vi "Arttu_v09_1.vi"() -> ()   [LabVIEW 2015]
panel:
  out "element":bool
  out "Started:":string
  in  "SHUTDOWN":bool
  in  "MASTER CONTROL":bool
  in  "Tab Control":T1(tab)
  in  "Read Seq":bool
  in  "Save Seq":bool
  in  "Configuration file":path=path "C:/Users/shresplab/Desktop/BerttaConfiguration.lvm" caption="Filename"
  in  "OK Button 2":bool
  out "Boolean":bool
  in  "User (initials)":string
  in  "Project name":string
  in  "Description":string
  out "Output file":string
  out "PUMP 3":bool
  out "Target amount":dbl
  out "Scale weight":dbl
  out "Amount now":dbl
  out "Flow rate":dbl
  out "Time to target":dbl format="%<%H:%M:%S>t"
  out "Current step":dbl
  out "Target amount":dbl
  out "Amount now":dbl
  out "Amount now":dbl
  out "Target amount":dbl
  out "Current step":dbl
  out "Time to target":dbl format="%<%H:%M:%S>t"
  out "Flow rate":dbl
  out "Amount now":dbl
  out "Scale weight":dbl
  out "Target amount":dbl
  out "PUMP 2":bool
  out "Sensor OK 6":bool
  out "Sensor OK 5":bool
  out "Sensor OK 4":bool
  out "Sensor OK 3":bool
  in  "OK Button":bool
  in  "Add comment":string
  out "PUMP 1":bool
  out "Target amount":dbl
  out "Scale weight":dbl
  out "Amount now":dbl
  out "Flow rate":dbl
  out "Time to target":dbl format="%<%H:%M:%S>t"
  out "Current step":dbl
  out "Target amount":dbl
  out "Amount now":dbl
  out "Tr":dbl
  out "Tj in":dbl
  out "Tj out":dbl
  out "T set":dbl
  out "Current step":i32
  out "RPM":dbl
  out "Torque 2":dbl
  out "Waveform Chart 5":dynamicdata(graph)
  out "Waveform Chart 6":dynamicdata(graph)
  out "Waveform Chart 7":dynamicdata(graph)
  in  "Tab Control 2":T2(tab)
  out "Waveform Chart 3":dynamicdata(graph)
  out "Waveform Chart 8":dynamicdata(graph)
  out "Waveform Chart 11":dynamicdata(graph)
  out "Waveform Chart 13":dynamicdata(graph)
  out "Waveform Chart 9":dynamicdata(graph)
  out "Table":string[][](table)=[["14.8.2017 18.06.59", "0,000000", "417,670000", "-0,150000", "1,000000", "22,220000", "23,366837", "23,574959", "23,985852", "23,690000", "240,000000", "4,000000", "0,000000", "397,000000", "-397,000000", "1,000000"], ["14.8.2017 18.07.06", "0,000000", "417,640000", "-0,120000", "1,000000", "22,220000", "23,763115", "23,906257", "23,985694", "23,680000", "240,000000", "4,000000", "0,000000", "397,000000", "-397,000000", "1,000000"], ["14.8.2017 18.07.13", "0,000000", "417,640000", "-0,120000", "1,000000", "22,220000", "23,965922", "24,013440", "23,984906", "23,670000", "240,000000", "4,100000", "3,000000", "397,000000", "-397,000000", "1,000000"], ["14.8.2017 18.07.21", "0,000000", "417,640000", "-0,120000", "1,000000", "22,220000", "23,943860", "23,900110", "23,987113", "23,670000", "240,000000", "4,000000", "0,000000", "397,000000", "-397,000000", "1,000000"], ["14.8.2017 18.07.28", "0,000000", "417,640000", "-0,120000", "1,000000", "22,220000", "23,736328", "23,600018", "23,989004", "23,660000", "240,000000", "4,000000", "0,000000", "397,000000", "-397,000000", "1,000000"], ["14.8.2017 18.07.36", "0,000000", "417,640000", "-0,120000", "1,000000", "22,220000", "23,480910", "23,324538", "23,991053", "23,660000", "240,000000", "4,000000", "0,000000", "397,000000", "-397,000000", "1,000000"], ["14.8.2017 18.07.43", "0,000000", "417,640000", "-0,120000", "2,000000", "22,220000", "23,195579", "23,008270", "23,999093", "23,650000", "240,000000", "4,000000", "0,000000", "397,000000", "-397,000000", "1,000000"], ["14.8.2017 18.07.51", "0,000000", "417,650000", "-417,650000", "1,000000", "22,220000", "22,862541", "22,649021", "24,003979", "23,650000", "240,000000", "4,000000", "0,000000", "397,000000", "-397,000000", "2,000000"], ["14.8.2017 18.07.58", "0,000000", "417,640000", "0,010000", "1,000000", "22,220000", "22,541353", "22,354878", "24,005398", "23,650000", "240,000000", "4,000000", "0,000000", "397,000000", "-397,000000", "1,000000"], ["14.8.2017 18.08.06", "0,000000", "417,640000", "0,010000", "1,000000", "22,220000", "22,347931", "22,253738", "24,007605", "23,640000", "240,000000", "4,100000", "0,000000", "397,000000", "-397,000000", "1,000000"], ["14.8.2017 18.08.13", "0,000000", "417,640000", "0,010000", "1,000000", "22,220000", "22,329030", "22,302102", "24,006028", "23,640000", "240,000000", "4,000000", "0,000000", "395,820000", "-395,820000", "1,000000"], ["14.8.2017 18.08.20", "0,000000", "417,640000", "0,010000", "1,000000", "22,220000", "22,466849", "22,511320", "24,002403", "23,630000", "240,000000", "4,000000", "0,000000", "395,830000", "-0,010000", "1,000000"], ["14.8.2017 18.08.28", "0,000000", "417,640000", "0,010000", "1,000000", "22,220000", "22,707062", "22,835101", "24,000984", "23,620000", "240,000000", "4,000000", "0,000000", "395,830000", "-0,010000", "1,000000"], ["14.8.2017 18.08.35", "0,000000", "417,640000", "0,010000", "1,000000", "22,220000", "23,054104", "23,232979", "24,001299", "23,600000", "240,000000", "4,000000", "0,000000", "395,830000", "-0,010000", "1,000000"], ["14.8.2017 18.08.43", "0,000000", "417,640000", "0,010000", "1,000000", "22,220000", "23,412371", "23,522793", "24,002560", "23,590000", "240,000000", "4,000000", "0,000000", "395,820000", "0,000000", "1,000000"], ["14.8.2017 18.08.51", "0,000000", "417,640000", "0,010000", "1,000000", "22,220000", "23,596247", "23,656125", "24,003821", "23,580000", "240,000000", "4,000000", "0,000000", "395,820000", "0,000000", "1,000000"]]
  in  "T ext / T ext 2":enum32{"External 1", "External 2"}(radio)
  out "Sensor OK":bool
  in  "T fail":dbl=20.0
  out "Boolean 12":bool
  out "Boolean 7":bool
  out "Boolean 6":bool
  out "Boolean 5":bool
  out "Boolean 4":bool
  in  "?":bool
  in  "T manual setpoint":dbl=20.0
  in  "Lauda port":dbl=9.0
  in  "Manual select":enum32{"Tr", "Tj"}(radio)
  in  "TempSeq":dbl[][](array[numeric])=[[20.0, 20.0, 0.0, 20.0], [20.0, 20.0, 0.0, 20.0], [50.0, 20.0, 0.0, 20.0], [20.0, 20.0, 0.0, 20.0], [20.0, 20.0, 0.0, 20.0], [20.0, 20.0, 1000.0, 20.0]]
  out "T control":dbl
  out "Tr":dbl
  out "Tj in":dbl
  out "Tj out":dbl
  out "DT":dbl
  out "Elapsed":i32 format="%<%H:%M:%S>T"
  in  "PAUSE":bool
  out "Boolean 19":bool
  in  "Reset":bool
  in  "Treshold (Tset)":dbl=1.0
  in  "Tmax":dbl=199.0
  in  "Tmin":dbl=20.0
  out "Waveform Chart":dynamicdata(graph)
  out "T external 2":dbl
  in  "Xe":dbl=1.0
  in  "Port":i32=10
  in  "Radio Buttons 3":enum32{"Reglo Digital", "Reglo Analog", "PAM"}(radio)=enum."Reglo Analog"
  out "Speed":dbl
  out "mA":dbl format="%#_2g"
  in  "Port":i32=15
  out "RPM":dbl format="%#_2g"
  out "Led10 3":bool
  out "Led9 3":bool
  out "Led8 3":bool
  out "Led7 3":bool
  out "Led6 3":bool
  out "Led5 3":bool
  out "Led4 3":bool
  out "Led3 3":bool
  out "Led2 3":bool
  out "Led1 3":bool
  in  "PumpSeq 3":dbl[][](array[numeric])=[[0.0, 0.0, 7.0], [0.0, 0.0, 2.0], [0.0, 0.0, 100.0], [0.0, 0.0, 0.0], [0.0, 0.0, 0.0], [0.0, 0.0, 0.0], [0.0, 0.0, 0.0], [0.0, 0.0, 0.0], [0.0, 0.0, 0.0], [0.0, 0.0, 0.0], [0.0, 1.0, 0.0]]
  in  "?":bool
  out "Flow rate (g/min)":dbl
  out "Scale reading":dbl
  out "Step amount now":dbl
  out "Time to target":dbl format="%<%H:%M:%S>t"
  in  "Grams / min":dbl
  out "Waveform Chart 12":dynamicdata(graph)
  in  "?":bool
  out "Total amount now":dbl
  out "Total time 3":dbl
  out "Total amount target 3":dbl
  out "Led11 3":bool
  in  "Reset 4":bool
  in  "Port":i32=11
  in  "Radio Buttons 2":enum32{"Reglo Digital", "Reglo Analog", "PAM"}(radio)
  out "Speed":dbl
  out "mA":dbl format="%#_2g"
  in  "Port":i32=15
  out "RPM":dbl format="%#_2g"
  out "Led10 2":bool
  out "Led9 2":bool
  out "Led8 2":bool
  out "Led7 2":bool
  out "Led6 2":bool
  out "Led5 2":bool
  out "Led4 2":bool
  out "Led3 2":bool
  out "Led2 2":bool
  out "Led1 2":bool
  in  "PumpSeq 2":dbl[][](array[numeric])=[[0.0, 0.0, 7.0], [0.0, 0.0, 2.0], [0.0, 0.0, 100.0], [0.0, 0.0, 0.0], [0.0, 0.0, 0.0], [0.0, 0.0, 0.0], [0.0, 0.0, 0.0], [0.0, 0.0, 0.0], [0.0, 0.0, 0.0], [0.0, 0.0, 0.0], [0.0, 1.0, 0.0]]
  in  "?":bool
  out "Flow rate (g/min)":dbl
  out "Scale reading":dbl
  out "Step amount now":dbl
  out "Time to target":dbl format="%<%H:%M:%S>t"
  in  "Grams / min":dbl
  out "Waveform Chart 10":dynamicdata(graph)
  in  "?":bool
  out "Total amount now":dbl
  out "Total time 2":dbl
  out "Total amount target 2":dbl
  out "Led11 2":bool
  in  "Reset 3":bool
  in  "Port":i32=12
  in  "Radio Buttons":enum32{"Reglo Digital", "Reglo Analog", "PAM"}(radio)
  out "Speed":dbl
  out "mA":dbl format="%#_2g"
  in  "Port":i32=14
  out "RPM":dbl format="%#_2g"
  out "Led10":bool
  out "Led9":bool
  out "Led8":bool
  out "Led7":bool
  out "Led6":bool
  out "Led5":bool
  out "Led4":bool
  out "Led3":bool
  out "Led2":bool
  out "Led1":bool
  in  "PumpSeq":dbl[][](array[numeric])=[[0.0, 0.0, 7.0], [0.0, 0.0, 2.0], [0.0, 0.0, 100.0], [0.0, 0.0, 0.0], [0.0, 0.0, 0.0], [0.0, 0.0, 0.0], [0.0, 0.0, 0.0], [0.0, 0.0, 0.0], [0.0, 0.0, 0.0], [0.0, 0.0, 0.0], [0.0, 1.0, 0.0]]
  in  "?":bool
  out "Flow rate (g/min)":dbl
  out "Scale reading":dbl
  out "Step amount now":dbl
  out "Time to target":dbl format="%<%H:%M:%S>t"
  in  "Grams / min":dbl
  out "Waveform Chart 2":dynamicdata(graph)
  in  "?":bool
  out "Total amount now":dbl
  out "Total time":dbl
  out "Total amount target":dbl
  out "Led11":bool
  in  "Reset 2":bool
  in  "Bypass select 2":enum32{"Remote", "Manual"}(radio)
  in  "Port":dbl=13.0
  out "RPM":dbl
  out "Torque":dbl
  in  "Set RPM":dbl(slide) scale=0.0..500.0
  out "Waveform Chart 4":dynamicdata(graph)
  in  "Adjust T":dbl
  in  "Cal pump 3":dbl=1.11
  in  "Cal pump 2":dbl=1.218 format="%#_13g"
  in  "Cal pump 1":dbl=1.0 format="%#_13g"
  out "DAQ 9217 (PT100)":errorcluster
  # "Temperature sensor:"
  # "Manual control:"
  # "PUMP & SCALE 1"
  # "STEP"
  # "TOTAL"
  # "PUMP & SCALE 2"
  # "STEP"
  # "TOTAL"
  # "PUMP & SCALE 3"
  # "STEP"
  # "TOTAL"
  # "Tinit     >    Tset          Wait            Tfail"
  # "Manual control / end of sequence"
  # "Manual control"
  # "Secondary temperature sensor"
  # "Device communication"
  # "Grams    /   min"
  # "End of sequence"
  # "Manual control"
  # "Device communication"
  # "Pump configuration"
  # "Scale configuration"
  # "SCALE 1"
  # "Grams    /   min"
  # "End of sequence"
  # "Manual control"
  # "Device communication"
  # "Pump configuration"
  # "Scale configuration"
  # "SCALE 2"
  # "Grams    /   min"
  # "End of sequence"
  # "Manual control"
  # "Device communication"
  # "Pump configuration"
  # "Scale configuration"
  # "SCALE 3"
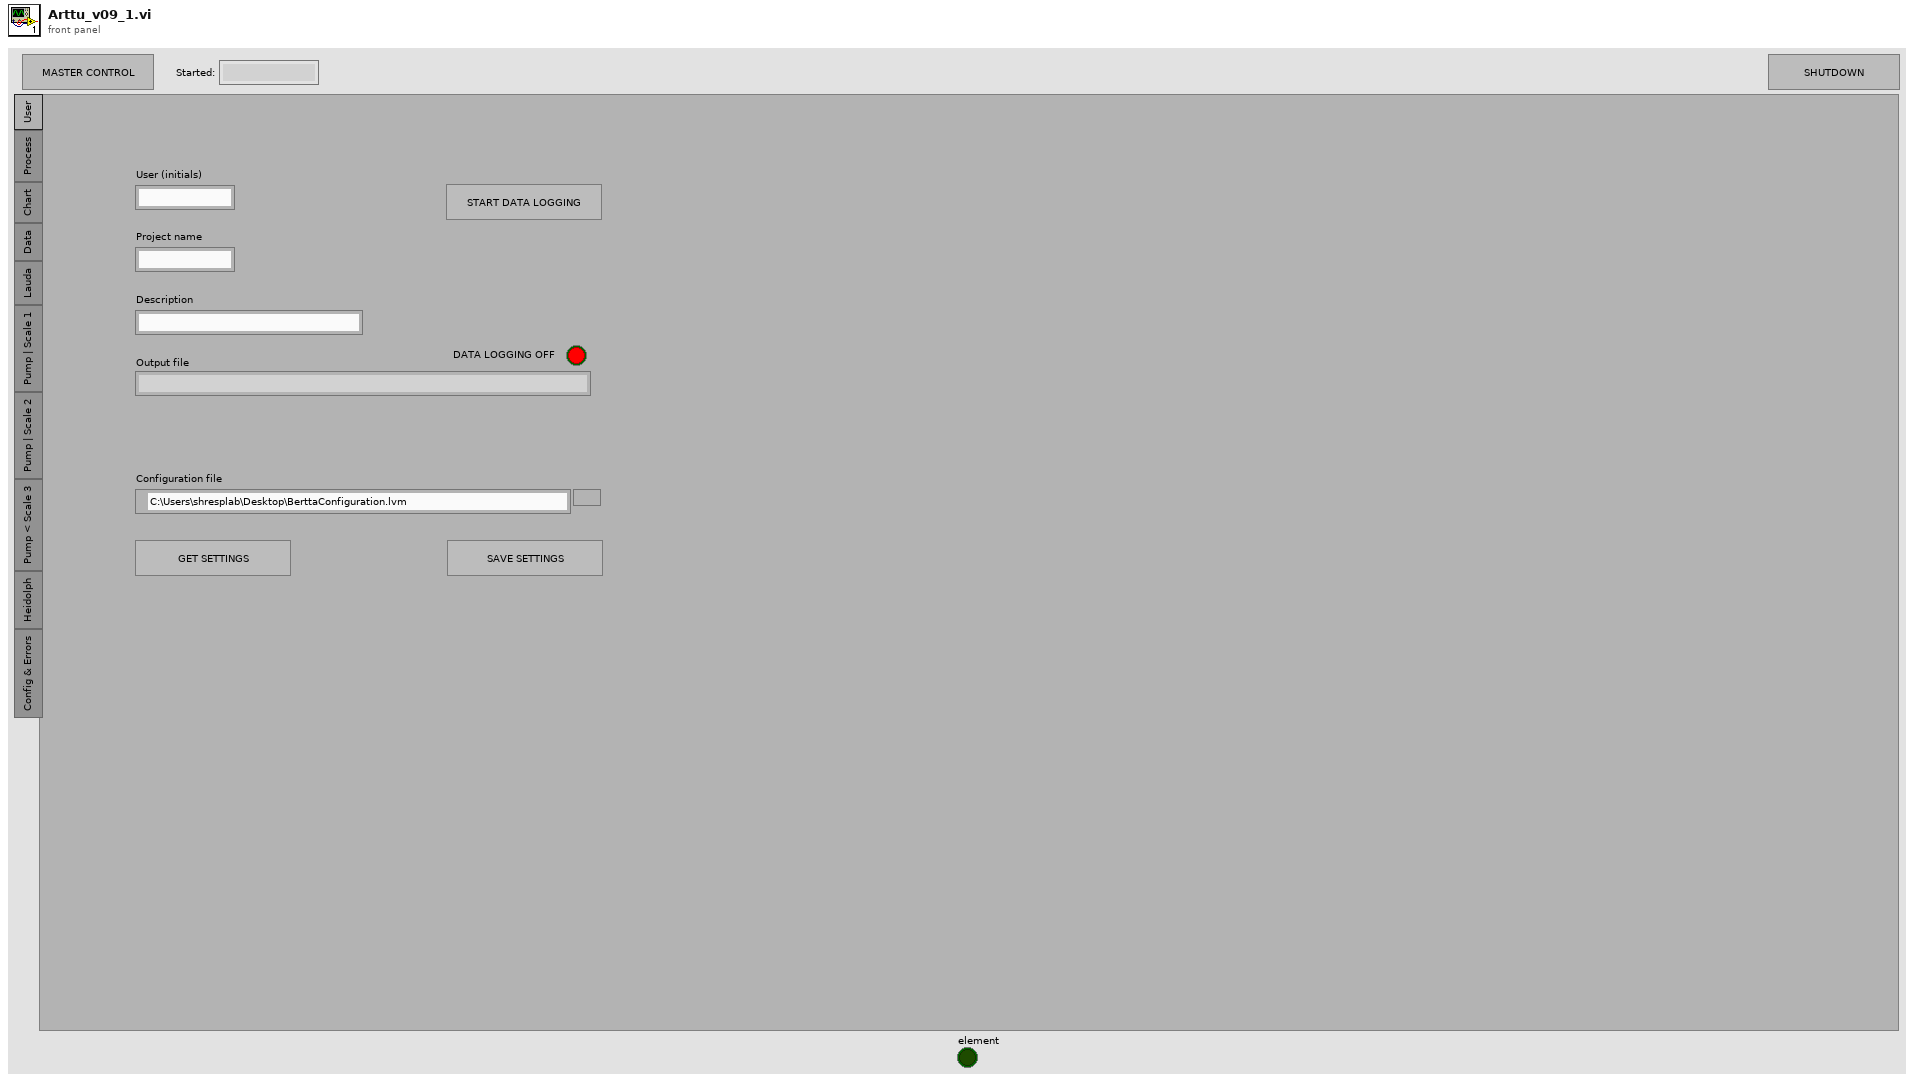
[diagram p1: front panel]
types:
  T1 = enum32{"User", "Process", "Chart", "Data", "Lauda", "Pump | Scale 1", "Pump | Scale 2", "Pump < Scale 3", "Heidolph", "Config & Errors"}
  T2 = enum32{"Temperatures", "Scale / Pump 1", "Scale / Pump 2", "Scale / Pump 3", "RPM / torque"}
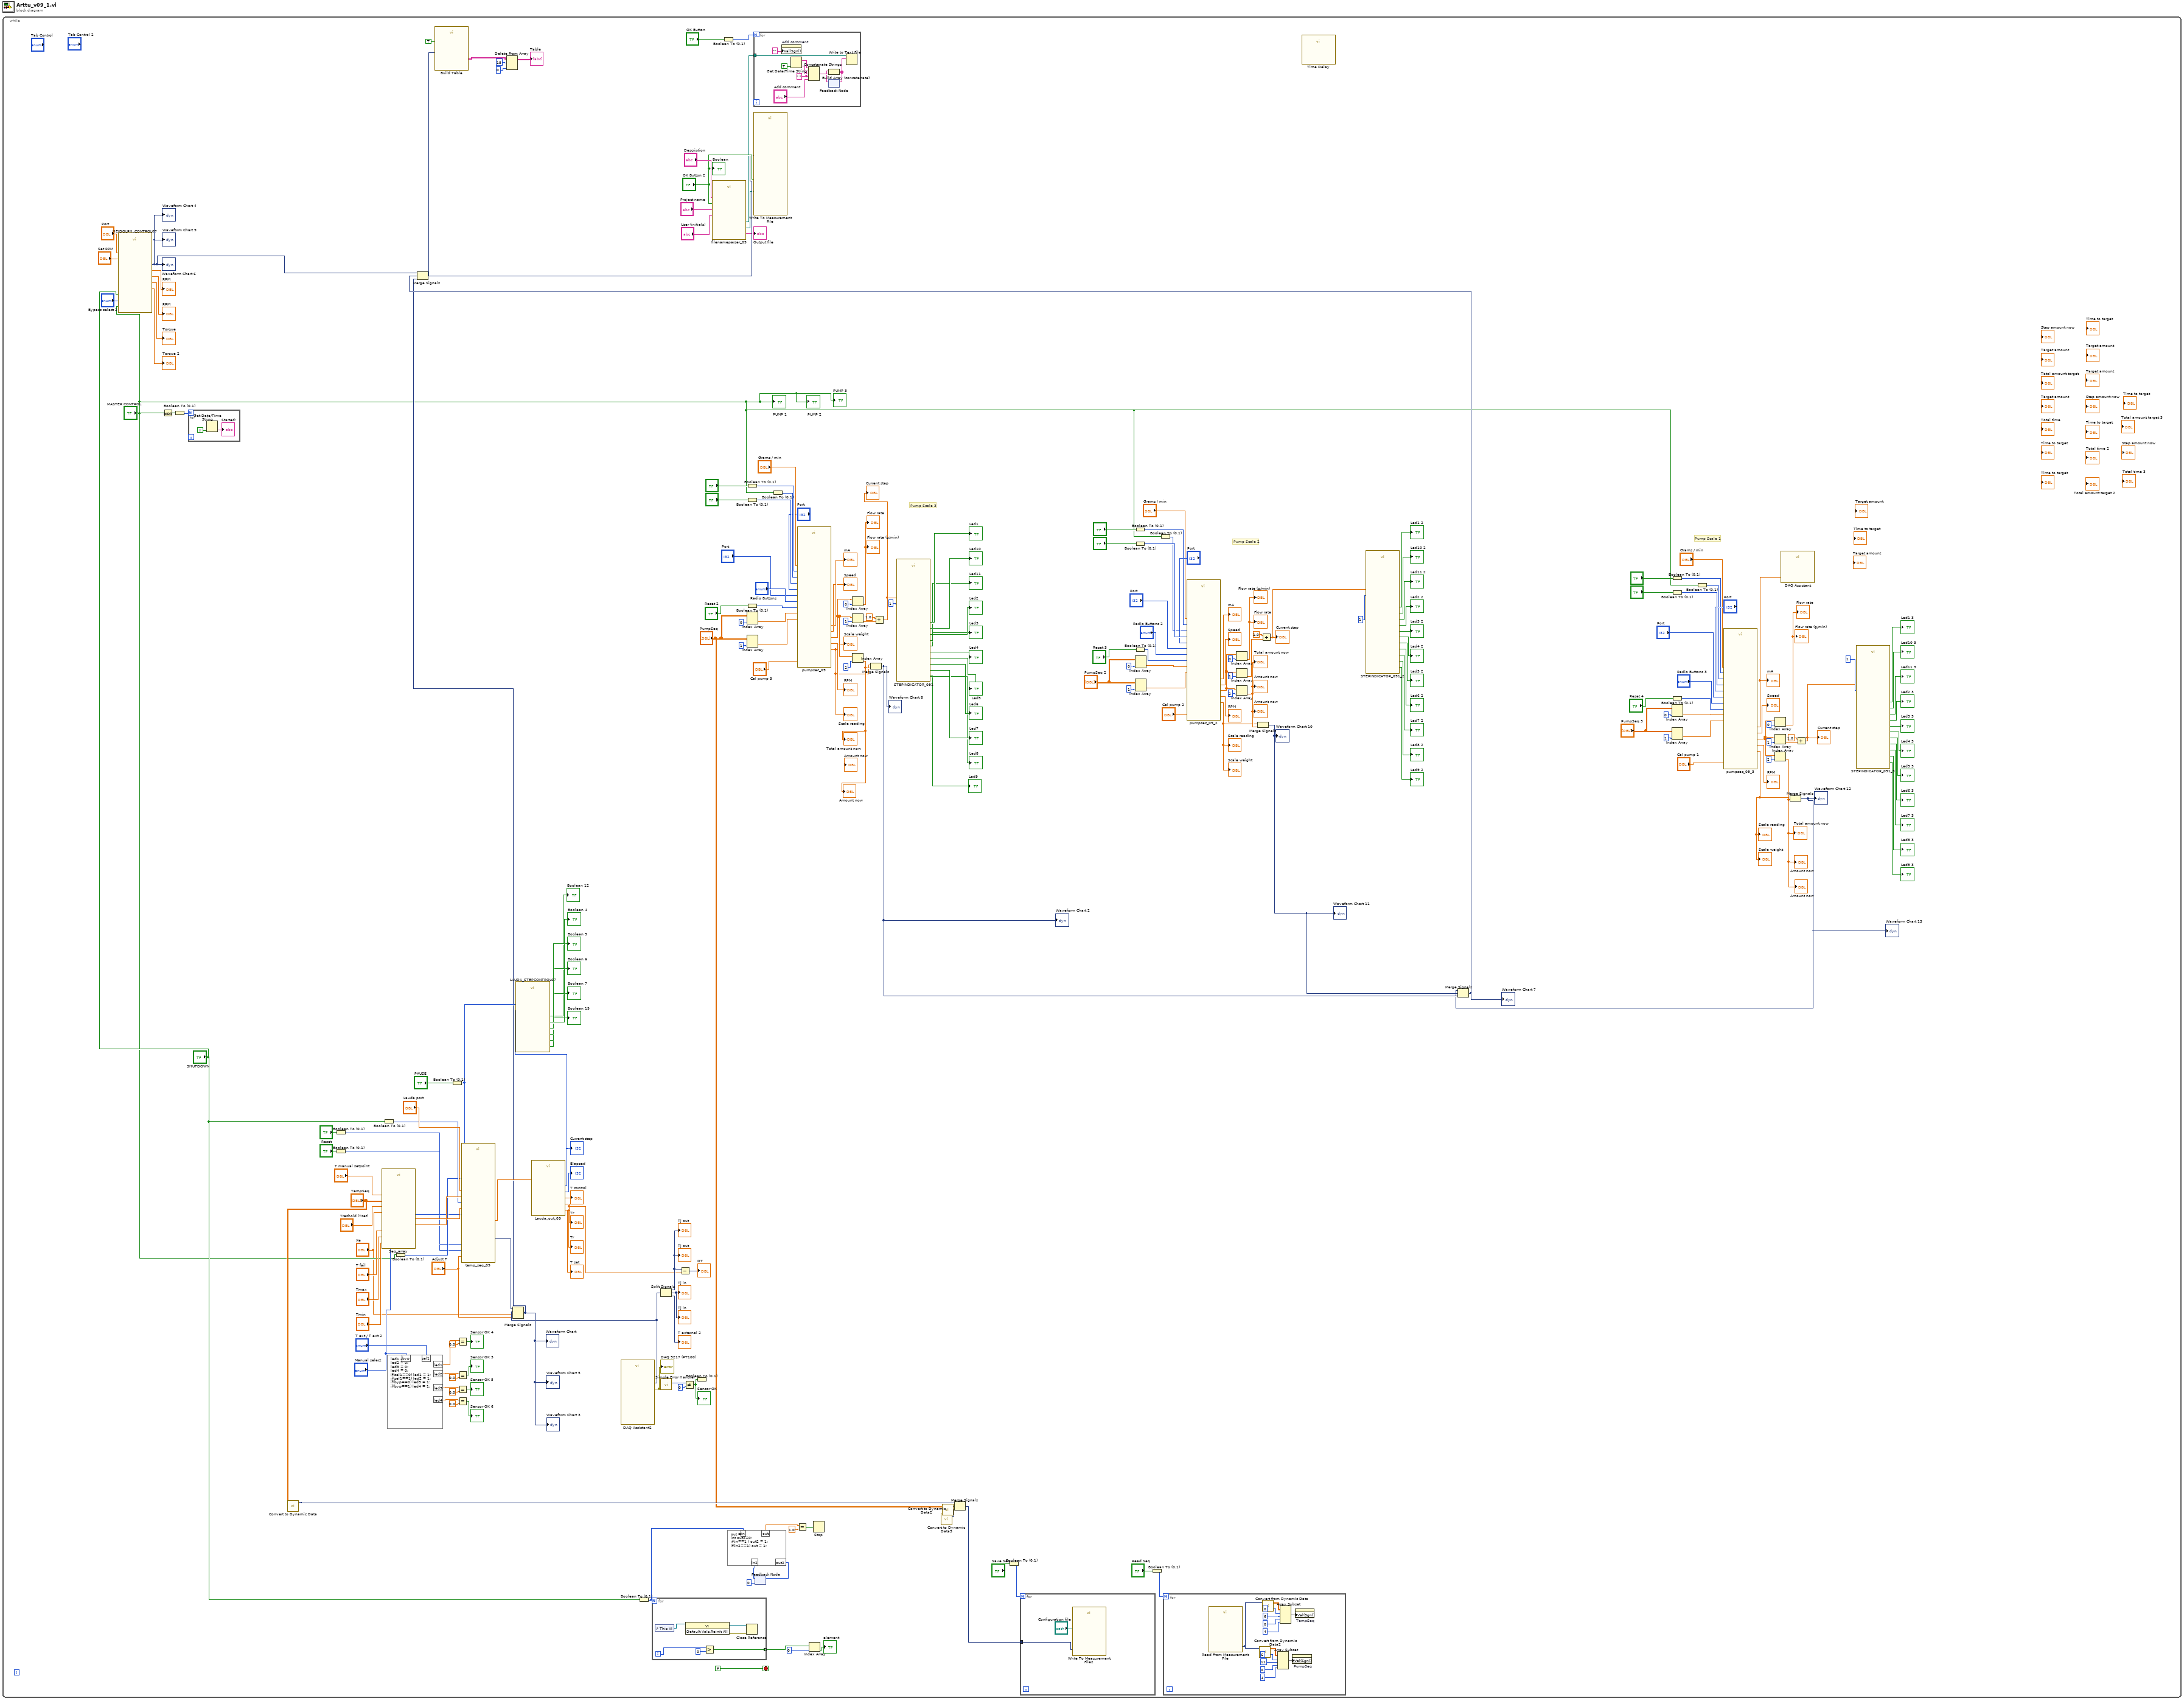
[diagram p0: block diagram]
diagram:
  n1 = while {
    stop <- FALSE stop-if-true
    # "Pump Scale 3"
    # "Pump Scale 2"
    # "Pump Scale 1"
    n2 = call "HEIDOLPH_CONTROL07.vi"("master"="MASTER CONTROL", "shutdown"="SHUTDOWN", "Bypass select"="Bypass select 2", "Set RPM"="Set RPM", "Device port"="Port") -> ("Dynamic Data"=w226:dynamicdata, "RPM"=→"RPM":dbl, "RPM 2"=→"RPM":dbl, "Torque"=→"Torque":dbl, "Torque 2"=→"Torque 2":dbl)  [unwired: 2 in]
    "Waveform Chart 4" <- w226
    "Waveform Chart 6" <- w226
    "Waveform Chart 9" <- w226
    n3 = Not(x="MASTER CONTROL") -> (.not. x?=w211:bool)
    n4 = Boolean To (0,1)(Boolean=w211) -> (0, 1=w212:i16)
    n5 = for {
      N: w212 -> [_]
      n6 = Get Date/Time String(want seconds? (F)=TRUE) -> (time string=→"Started:":string)  [unwired: 2 in, 1 out]
    }
    n7 = call "Convert to Dynamic Data"("2D Array"="TempSeq") -> ("Dynamic Data Type"=w208:dynamicdata)  [unwired: 3 in]
    n8 = Boolean To (0,1)(Boolean="Reset") -> (0, 1=w150:i16)
    n9 = Boolean To (0,1)(Boolean="?") -> (0, 1=w152:i16)
    n10 = call "Seq_array.vi"("Tfail_manual"="T fail", "TempSeq in"="TempSeq", "Tmin"="Tmin", "Tmax"="Tmax", "Treshold (Tset)"="Treshold (Tset)", "T manual setpoint"="T manual setpoint", "Xe"="Xe") -> ("TimeParams"=w164:dbl[], "TempParams"=w165:dbl[])  [unwired: 3 in]
    n11 = Boolean To (0,1)(Boolean="SHUTDOWN") -> (0, 1=w160:i16)
    n12 = formula code="led1 = 0;\nled2 = 0;\nled3 = 0;\nled4 = 0;\nif(sel1==0) led1 = 1;\nif(sel1==1) led2 = 1;\nif(byp==0) led3 = 1;\nif(byp==1) led4 = 1;"("sel1"="T ext / T ext 2", "byp"="Manual select") -> ("led1"=w179:dbl, "led2"=w177:dbl, "led3"=w172:dbl, "led4"=w171:dbl)
    n13 = Boolean To (0,1)(Boolean="MASTER CONTROL") -> (0, 1=w159:i16)
    n14 = Boolean To (0,1)(Boolean="PAUSE") -> (0, 1=w156:i16)
    n15 = Equal?(x=w179, y=0.0) -> (x = y?=→"Sensor OK 4":bool)
    n16 = Equal?(x=w177, y=0.0) -> (x = y?=→"Sensor OK 3":bool)
    n17 = Equal?(x=w172, y=0.0) -> (x = y?=→"Sensor OK 5":bool)
    n18 = Equal?(x=w171, y=0.0) -> (x = y?=→"Sensor OK 6":bool)
    n19 = call "temp_seq_09.vi"("master"=w159, "shutdown"=w160, "Tr_orTj"="Manual select", "pause"=w156, "adjust"="Adjust T", "TempParams"=w165, "TimeParams"=w164, "port"="Lauda port", "reset"=w150, "manual"=w152) -> ("params"=w157:dbl[], "Waveform Chart"=w21:dynamicdata)  [unwired: 2 in, 2 out]
    n20 = call "Lauda_out_09.vi"("params"=w157) -> ("Elapsed"=→"Elapsed":i32, "Tr"=w19:dbl, "Current step"=w141:i32, "T control"=→"T control":dbl, "T set"=→"T set":dbl)  [unwired: 6 in]
    "Tr" <- w19
    "Tr" <- w19
    "Current step" <- w141
    n21 = call "LAUDA_STEPCONTROL07.vi"("step"=w141, "pause"=w156) -> ("Boolean 13"=→"Boolean 19":bool, "Boolean 6"=→"Boolean 6":bool, "Boolean 5"=→"Boolean 5":bool, "Boolean 4"=→"Boolean 4":bool, "Boolean 7"=→"Boolean 7":bool, "Boolean 12"=→"Boolean 12":bool)  [unwired: 4 in]
    n22 = call "DAQ Assistant2"() -> ("data"=w20:dynamicdata, "error out"=w221:errorcluster)  [unwired: 17 in, 1 out]
    "DAQ 9217 (PT100)" <- w221
    n23 = Merge Signals(w21, w20, "Xe", "Adjust T") -> (w16:dynamicdata)
    "Waveform Chart 3" <- w16
    "Waveform Chart" <- w16
    "Waveform Chart 5" <- w16
    n24 = Boolean To (0,1)(Boolean="SHUTDOWN") -> (0, 1=w185:i16)
    n25 = for {
      N: w185 -> [_]
      tunnel: [w258] -> w210 mode=indexing
      i -> [w260]
      n26 = control-ref of="This VI"() -> (w263:refnum<vi>)
      n27 = invoke class="VI" method="Default Vals.Reinit All"(reference=w263) -> (reference out=w261:refnum<vi>, error out=w262:errorcluster)  [unwired: 2 in, 1 out]
      n28 = Greater?(x=w260, y=0) -> (0:w258:bool)
      n29 = Close Reference(reference=w261, error in (no error)=w262) -> ()  [unwired: 1 out]
    }
    n30 = Split Signals(w20) -> (w143:dynamicdata, →"Tj in" →"Tj in":dynamicdata, →"T external 2":dynamicdata)  [unwired: 3 in]
    "Tj out" <- w143
    "Tj out" <- w143
    n31 = call <vilib>:"Simple Error Handler.vi"("error in (no error)"=w221) -> ("code out"=w220:i32)  [unwired: 4 in, 4 out]
    n32 = Subtract(x=w143, y=w19) -> (x-y=→"DT":dynamicdata)
    n33 = Not Equal?(x=w220, y=0) -> (x != y?=w201:bool)
    "Sensor OK" <- w201
    n34 = Boolean To (0,1)(Boolean=w201) -> ()  [unwired: 1 out]
    n35 = call "filenameparser_09.vi"("Description"="Description", "Project name"="Project name", "User (initials)"="User (initials)", "OK Button in"="OK Button 2") -> ("Output file"=→"Output file":string, "appended path 2"=w192:path, "appended path"=w191:path)  [unwired: 5 in]
    n36 = Boolean To (0,1)(Boolean="OK Button") -> (0, 1=w190:i16)
    n37 = Boolean To (0,1)(Boolean="?") -> (0, 1=w132:i16)
    n38 = Boolean To (0,1)(Boolean="?") -> (0, 1=w128:i16)
    n39 = Boolean To (0,1)(Boolean="Reset 2") -> (0, 1=w130:i16)
    n40 = Index Array(array="PumpSeq", index (col)=0 ("disabled index (col)")) -> (element=w137:dbl[])  [unwired: 1 in]
    n41 = Index Array(array="PumpSeq", index (col)=1 ("disabled index (col)")) -> (element=w136:dbl[])  [unwired: 1 in]
    n42 = for {
      N: w190 -> [_]
      tunnel: w191 -> [w235]
      w239 = " " ("string")
      n43 = property on="Add comment" class="Str"("Val(Sgnl)"="" ("Value (Signaling)")) -> ()  [unwired: 2 in, 2 out]
      n44 = Get Date/Time String(want seconds? (F)=TRUE) -> (date string=w242:string, time string=w240:string)  [unwired: 2 in]
      n45 = Concatenate Strings(w242, w239, w240, w239, "Add comment") -> (w238:string)
      n46 = feedback #1() -> (w237:string[])  [unwired: 1 in]
      n47 = Build Array (concatenate)(w237, w238) -> (w236:string[])
      n48 = feedback-in #1(w236) -> ()
      n49 = Write to Text File(file (use dialog)=w235, text=w236) -> ()  [unwired: 2 in, 3 out]
    }
    n50 = feedback #2(0) -> (w183:i32)
    n51 = formula code="out = 0;\nint out2=0;\nif(in==1 ) out2 = 1;\nif(in2==1) out = 1;"("in"=w185, "in2"=w183) -> ("out"=w187:dbl, "out2"=w184:i32)
    n52 = feedback-in #2(w184) -> ()
    n53 = Boolean To (0,1)(Boolean="MASTER CONTROL") -> (0, 1=w127:i16)
    n54 = Equal?(x=w187, y=1.0) -> (x = y?=w186:bool)
    n55 = call "pumpsec_09.vi"("reset"=w130, "master"=w127, "correction"="Cal pump 3", "manual"=w132, "pause"=w128, "Port"="Port", "pump_type"="Radio Buttons", "port, Reglo D"="Port", "Target"=w137, "Time"=w136, "fr_manual"="Grams / min") -> ("Reglo D"=→"RPM":dbl, "Scale"=w60:dbl, "mA"=→"mA":dbl, "params"=w119:dbl[], "PAM"=→"Speed":dbl)  [unwired: 3 in, 1 out]
    "Scale reading" <- w60
    "Scale weight" <- w60
    n56 = Index Array(array=w210, index=0) -> (element=→"element":bool)
    n57 = Stop(stop? (T)=w186) -> ()
    n58 = Index Array(array=w119, index=0) -> (element=→"Flow rate (g/min)" →"Flow rate":dbl)
    n59 = Index Array(array=w119, index=1) -> (element=w121:dbl)
    n60 = Index Array(array=w119, index=2) -> (element=w101:dbl)
    "Total amount now" <- w101
    "Amount now" <- w101
    n61 = Merge Signals(w60, w101) -> (w18:dynamicdata)
    "Waveform Chart 2" <- w18
    "Waveform Chart 8" <- w18
    n62 = Add(x=1.0, y=w121) -> (x+y=w103:dbl)
    "Current step" <- w103
    n63 = call "STEPINDICATOR_091.vi"("current step"=w103, "enable"=i16 1) -> ("Led 8"=→"Led8":bool, "Led 10"=→"Led10":bool, "Led 11"=→"Led11":bool, "Led 7"=→"Led7":bool, "Led 1"=→"Led1":bool, "Led 6"=→"Led6":bool, "Led 2"=→"Led2":bool, "Led 5"=→"Led5":bool, "Led 4"=→"Led4":bool, "Led 3"=→"Led3":bool, "Led 9"=→"Led9":bool)  [unwired: 3 in]
    n64 = call "Convert to Dynamic Data3"() -> ("Dynamic Data Type"=w168:dynamicdata)  [unwired: 4 in]
    n65 = call "Convert to Dynamic Data2"("2D Array"="PumpSeq") -> ("Dynamic Data Type"=w207:dynamicdata)  [unwired: 3 in]
    n66 = Merge Signals(w208, w207, w168) -> (w206:dynamicdata)
    n67 = Boolean To (0,1)(Boolean="Save Seq") -> (0, 1=w205:i16)
    n68 = for {
      N: w205 -> [_]
      tunnel: w206 -> [w257]
      n69 = call "Write To Measurement File2"("Signals"=w257, "Filename"="Configuration file") -> ()  [unwired: 15 in, 3 out]
    }
    n70 = Boolean To (0,1)(Boolean="?") -> (0, 1=w83:i16)
    n71 = Boolean To (0,1)(Boolean="?") -> (0, 1=w94:i16)
    n72 = Boolean To (0,1)(Boolean="Reset 3") -> (0, 1=w90:i16)
    n73 = Index Array(array="PumpSeq 2", index (col)=0 ("disabled index (col)")) -> (element=w97:dbl[])  [unwired: 1 in]
    n74 = Index Array(array="PumpSeq 2", index (col)=1 ("disabled index (col)")) -> (element=w96:dbl[])  [unwired: 1 in]
    n75 = Boolean To (0,1)(Boolean="Read Seq") -> (0, 1=w202:i16)
    n76 = Boolean To (0,1)(Boolean="MASTER CONTROL") -> (0, 1=w81:i16)
    n77 = for {
      N: w202 -> [_]
      n78 = call "Read From Measurement File"() -> ("Signals"=w245:dynamicdata)  [unwired: 6 in, 5 out]
      n79 = call "Convert from Dynamic Data2"("Dynamic Data Type"=w245) -> ("Array"=w244:dbl[][])  [unwired: 3 in]
      n80 = call "Convert from Dynamic Data"("Dynamic Data Type"=w245) -> ("Array"=w253:dbl[][])  [unwired: 3 in]
      n81 = Array Subset(array=w244, index (row)=6 ("index"), length (row)=11 ("length"), index (col)=0 ("index"), length (col)=4 ("length")) -> (w243:dbl[][])
      n82 = Array Subset(array=w253, index (row)=0 ("index"), length (row)=6 ("length"), index (col)=0 ("index"), length (col)=4 ("length")) -> (w250:dbl[][])
      n83 = property on="PumpSeq" class="Arr (strict)"("Val(Sgnl)"=w243) -> ()  [unwired: 2 in, 2 out]
      n84 = property on="TempSeq" class="Arr (strict)"("Val(Sgnl)"=w250) -> ()  [unwired: 2 in, 2 out]
    }
    n85 = call "pumpsec_09_2.vi"("reset"=w90, "master"=w81, "correction"="Cal pump 2", "manual"=w83, "pause"=w94, "Port"="Port", "pump_type"="Radio Buttons 2", "port, Reglo D"="Port", "Target"=w97, "fr_manual"="Grams / min", "Time"=w96) -> ("Reglo D"=→"RPM":dbl, "Scale"=w61:dbl, "mA"=→"mA":dbl, "params"=w84:dbl[], "PAM"=→"Speed":dbl)  [unwired: 3 in, 1 out]
    "Scale weight" <- w61
    "Scale reading" <- w61
    n86 = Index Array(array=w84, index=0) -> (element=→"Flow rate" →"Flow rate (g/min)":dbl)
    n87 = Index Array(array=w84, index=1) -> (element=w87:dbl)
    n88 = Index Array(array=w84, index=2) -> (element=w62:dbl)
    "Amount now" <- w62
    "Amount now" <- w62
    "Total amount now" <- w62
    n89 = Merge Signals(w61, w62) -> (w17:dynamicdata)
    "Waveform Chart 11" <- w17
    "Waveform Chart 10" <- w17
    n90 = Add(x=1.0, y=w87) -> (x+y=w74:dbl)
    "Current step" <- w74
    n91 = call "Time Delay"() -> ()  [unwired: 11 in, 1 out]
    n92 = call "STEPINDICATOR_091_2.vi"("current step"=w74, "enable"=i16 1) -> ("Led 8"=→"Led8 2":bool, "Led 10"=→"Led10 2":bool, "Led 11"=→"Led11 2":bool, "Led 7"=→"Led7 2":bool, "Led 1"=→"Led1 2":bool, "Led 6"=→"Led6 2":bool, "Led 2"=→"Led2 2":bool, "Led 5"=→"Led5 2":bool, "Led 4"=→"Led4 2":bool, "Led 3"=→"Led3 2":bool, "Led 9"=→"Led9 2":bool)  [unwired: 3 in]
    n93 = Boolean To (0,1)(Boolean="?") -> (0, 1=w53:i16)
    n94 = Boolean To (0,1)(Boolean="?") -> (0, 1=w39:i16)
    n95 = Boolean To (0,1)(Boolean="Reset 4") -> (0, 1=w25:i16)
    n96 = Index Array(array="PumpSeq 3", index (col)=0 ("disabled index (col)")) -> (element=w48:dbl[])  [unwired: 1 in]
    n97 = Index Array(array="PumpSeq 3", index (col)=1 ("disabled index (col)")) -> (element=w47:dbl[])  [unwired: 1 in]
    n98 = Boolean To (0,1)(Boolean="MASTER CONTROL") -> (0, 1=w52:i16)
    n99 = call "pumpsec_09_3.vi"("reset"=w25, "master"=w52, "correction"="Cal pump 1", "manual"=w53, "pause"=w39, "Port"="Port", "pump_type"="Radio Buttons 3", "port, Reglo D"="Port", "Target"=w48, "fr_manual"="Grams / min", "Time"=w47) -> ("Reglo D"=→"RPM":dbl, "Scale"=w11:dbl, "mA"=w24:dbl, "params"=w44:dbl[], "PAM"=→"Speed":dbl)  [unwired: 3 in, 1 out]
    "Scale reading" <- w11
    "mA" <- w24
    "Scale weight" <- w11
    n100 = Index Array(array=w44, index=0) -> (element=→"Flow rate (g/min)" →"Flow rate":dbl)
    n101 = Index Array(array=w44, index=1) -> (element=w46:dbl)
    n102 = Index Array(array=w44, index=2) -> (element=w13:dbl)
    "Total amount now" <- w13
    "Amount now" <- w13
    "Amount now" <- w13
    n103 = call "DAQ Assistant"("data"=w24) -> ()  [unwired: 17 in, 2 out]
    n104 = Merge Signals(w11, w13) -> (w15:dynamicdata)
    "Waveform Chart 12" <- w15
    "Waveform Chart 13" <- w15
    n105 = Merge Signals(w15, w17, w18) -> (w22:dynamicdata)
    "Waveform Chart 7" <- w22
    n106 = Merge Signals(w226, w22, w16) -> (w197:dynamicdata)
    n107 = call "Build Table"("Include time data"=TRUE, "Signals"=w197) -> ("Table"=w196:string[][])  [unwired: 3 in, 6 out]
    n108 = Delete From Array(array=w196, length=15, index (col)=0 ("index (row)")) -> (array with subset deleted=→"Table":string[][])  [unwired: 1 in, 1 out]
    n109 = call "Write To Measurement File"("Signals"=w197, "Enable"="OK Button 2", "Filename"=w192) -> ()  [unwired: 14 in, 3 out]
    n110 = Add(x=1.0, y=w46) -> (x+y=w12:dbl)
    "Current step" <- w12
    n111 = call "STEPINDICATOR_091_3.vi"("current step"=w12, "enable"=i16 1) -> ("Led 8"=→"Led8 3":bool, "Led 10"=→"Led10 3":bool, "Led 11"=→"Led11 3":bool, "Led 7"=→"Led7 3":bool, "Led 1"=→"Led1 3":bool, "Led 6"=→"Led6 3":bool, "Led 2"=→"Led2 3":bool, "Led 5"=→"Led5 3":bool, "Led 4"=→"Led4 3":bool, "Led 3"=→"Led3 3":bool, "Led 9"=→"Led9 3":bool)  [unwired: 3 in]
    "PUMP 1" <- "MASTER CONTROL"
    "Boolean" <- "OK Button 2"
    "PUMP 2" <- "MASTER CONTROL"
    "PUMP 3" <- "MASTER CONTROL"
  }
